vi "PrepareDataToGraph.vi"(8 "Error In":errorcluster, 10 "GreyLevel Drops and time":dbl[][](array[numeric]), 11 "Rel Time (s)":u32[](array[numeric])) -> (0 "Error Out":errorcluster, 3 "Graph XY data":cluster{u32[], "GreyLevelArray":dbl[]}[](array[cluster]))   [LabVIEW 2015]
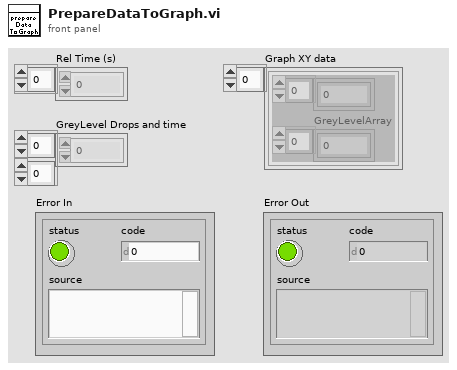
[diagram p1: front panel]
types:
  T1 = cluster{"Rel Time (s)":u32[], "GreyLevel Drops and time":dbl[]}
  T2 = cluster{"Rel Time (s)":u32[], "GreyLevel Drops and time":dbl[]}[]
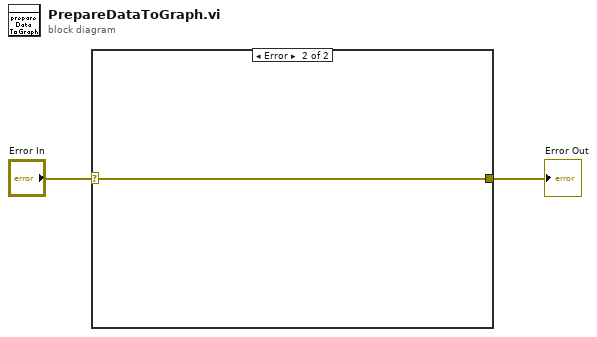
[diagram p0: block diagram]
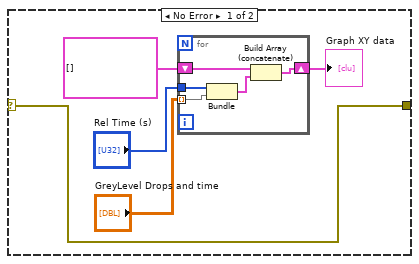
[diagram p2: hidden frame]
diagram:
  n1 = case shown="Error" "Error In" {
    selector: "Error In" -> [w3 w13]
    tunnel: [w3 w13] -> w1
    frame No Error {
      n2 = for {
        tunnel: "Rel Time (s)" -> [w12]
        tunnel: "GreyLevel Drops and time" -> [w11] mode=indexing
        shift-right: [w9] -> w5
        shift-left: cluster{u32[], "GreyLevelArray":dbl[]}[] [] -> [w8]
        n3 = Bundle("Rel Time (s)"=w12, "GreyLevel Drops and time"=w11) -> (w10:T1)  [unwired: 1 in]
        n4 = Build Array (concatenate)(w8, w10) -> (w9:T2)
      }
      "Graph XY data" <- w5
    }
    frame Error {
    }
  }
  "Error Out" <- w1
